vi "sub UI get b.vi"(8 "error in (no error)":errorcluster, 11 "IDE simple in":refnum<class "LF2R IDE.lvclass">) -> (0 "error out":errorcluster, 1 "<b> data":T1, 2 "index":u32, 3 "IDE simple out":refnum<class "LF2R IDE.lvclass">)   [LabVIEW 2018, in "LF2R IDE.lvlib" / "LF2R IDE.lvclass"]
uses:
  LF2R IDE.lvclass
  Frame Analizer/frame b data.ctl
  LF2R IDE.lvclass/LF2R IDE.ctl
  Frame Analizer/Data Parser.lvclass
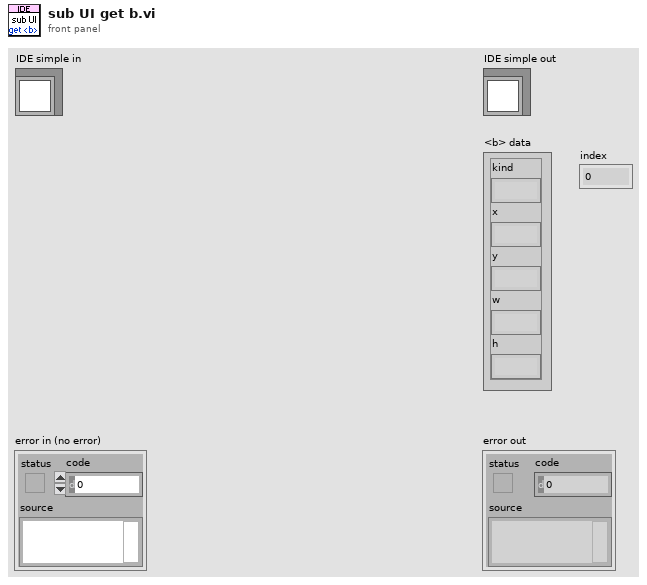
[diagram p1: front panel]
types:
  T1 = typedef "Data Parser.lvclass/frame b data.ctl" = cluster{"kind":string, "x":string, "y":string, "w":string, "h":string}
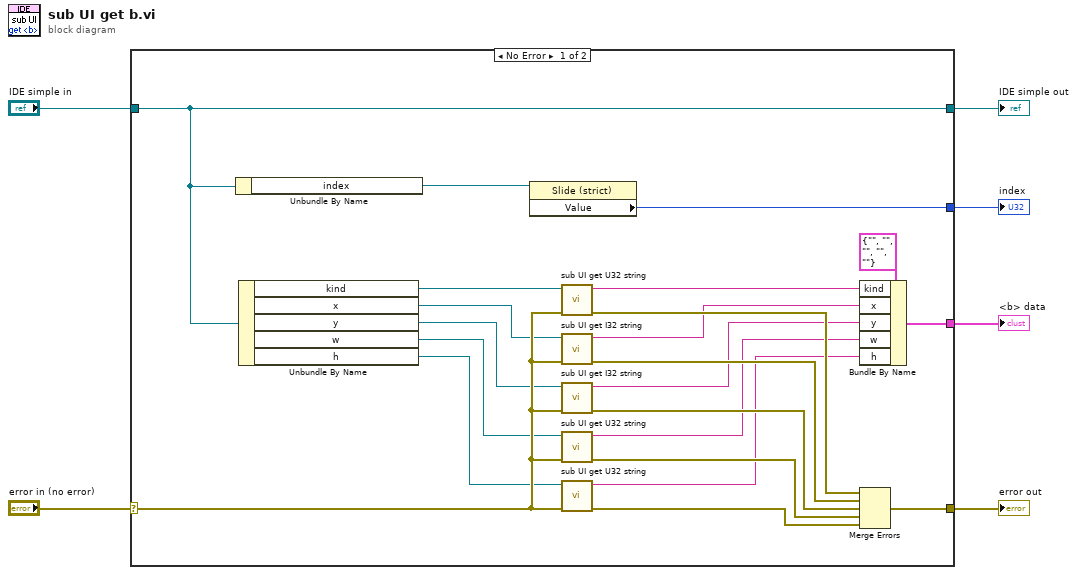
[diagram p0: block diagram]
diagram:
  n1 = case shown="No Error" "error in (no error)" {
    selector: "error in (no error)" -> [w24 w30]
    tunnel: [w27 w30] -> w5
    tunnel: [w13 w29] -> w3
    tunnel: "IDE simple in" -> [w13 w29]
    tunnel: [w26 _] -> w2
    tunnel: [w11 _] -> w1
    frame No Error {
      n2 = Unbundle By Name(w13) -> ("index"=w12:refnum<vi>)
      n3 = Unbundle By Name(w13) -> ("kind"=w25:refnum<vi>, "x"=w10:refnum<vi>, "y"=w9:refnum<vi>, "w"=w8:refnum<vi>, "h"=w7:refnum<vi>)
      n4 = property class="Slide (strict)"(reference=w12) -> ("Value"=w11:u32)  [unwired: 1 in, 2 out]
      n5 = call "sub UI get U32 string.vi"("error in (no error)"=w24, "U32 Ref"=w25) -> ("error out"=w23:errorcluster, "Value string"=w18:string)  [unwired: 8 in]
      n6 = call "sub UI get I32 string.vi"("error in (no error)"=w24, "I32 Ref"=w10) -> ("error out"=w22:errorcluster, "Value string"=w17:string)  [unwired: 8 in]
      n7 = call "sub UI get I32 string.vi"("error in (no error)"=w24, "I32 Ref"=w9) -> ("error out"=w21:errorcluster, "Value string"=w16:string)  [unwired: 8 in]
      n8 = call "sub UI get U32 string.vi"("error in (no error)"=w24, "U32 Ref"=w8) -> ("error out"=w20:errorcluster, "Value string"=w15:string)  [unwired: 8 in]
      n9 = call "sub UI get U32 string.vi"("error in (no error)"=w24, "U32 Ref"=w7) -> ("error out"=w19:errorcluster, "Value string"=w14:string)  [unwired: 8 in]
      n10 = Bundle By Name(cluster=T1 {"kind"="", "x"="", "y"="", "w"="", "h"=""} ("<b> data 2"), "kind"=w18, "x"=w17, "y"=w16, "w"=w15, "h"=w14) -> (w26:T1)
      n11 = Merge Errors(w23, w22, w21, w20, w19) -> (w27:errorcluster)
    }
    frame Error {
    }
  }
  "error out" <- w5
  "IDE simple out" <- w3
  "<b> data" <- w2
  "index" <- w1
